vi "Drive Train Code Stuff.vi"(8 "error in (no error)":errorcluster, 11 "RobotDriveDevRef":T1) -> ()   [LabVIEW 2012]
uses:
  <vilib>/Rock Robotics/WPI/RobotDrive/WPI_RobotDriveDevRef.ctl
  <vilib>/Rock Robotics/WPI/MotorControl/WPI_MotorControlDeviceRef.ctl
  <vilib>/Rock Robotics/SystemInterfaces/Typedef/FPGA_TypedefDigitalModule.ctl
  <vilib>/Rock Robotics/SystemInterfaces/DIO/FPGA_DIOPWMChannel.ctl
  <vilib>/Rock Robotics/WPI/PWM/WPI_PWMDeadband.ctl
  <vilib>/Rock Robotics/WPI/CAN/Jaguar/SubVIs/WPI_CANJaguar_ControlMode.ctl
  <vilib>/Rock Robotics/WPI/PWM/WPI_PWMTransform_ConPane.ctl
  Robot Global Data.vi
  Documents/LabVIEW Data/No Wayne Drive/wayne drive.vi
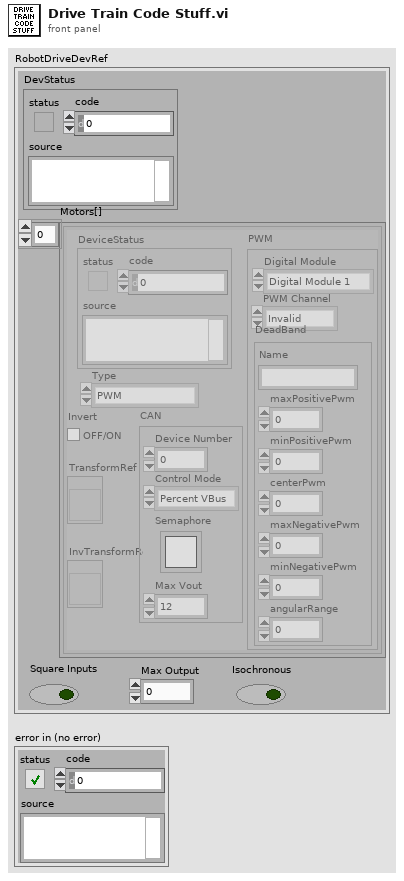
[diagram p1: front panel]
types:
  T1 = typedef "WPI_RobotDriveDevRef.ctl" = cluster{"DevStatus":errorcluster, "Motors[]":T2[], "Square Inputs":bool, "Max Output":dbl, "Isochronous":bool}
  T2 = typedef "WPI_MotorControlDeviceRef.ctl" = cluster{"DeviceStatus":errorcluster, "Type":enum16{"PWM", "CAN"}, "PWM":cluster{"Digital Module":T3, "PWM Channel":T4, "DeadBand":T5}, "CAN":cluster{"Device Number":u8, "Control Mode":T6, "Semaphore":T7, "Max Vout":dbl}, "Invert":bool, "TransformRef":T8, "InvTransformRef":T8}
  T3 = typedef "FPGA_TypedefDigitalModule.ctl" = enum16{"Digital Module 1", "Digital Module 2"}
  T4 = typedef "FPGA_DIOPWMChannel.ctl" = enum8{"PWM 1", "PWM 2", "PWM 3", "PWM 4", "PWM 5", "PWM 6", "PWM 7", "PWM 8", "PWM 9", "PWM 10", "Invalid"}
  T5 = typedef "WPI_PWMDeadband.ctl" = cluster{"Name":string, "maxPositivePwm":i32, "minPositivePwm":i32, "centerPwm":i32, "maxNegativePwm":i32, "minNegativePwm":i32, "angularRange":u16}
  T6 = typedef "WPI_CANJaguar_ControlMode.ctl" = enum8{"Percent VBus", "Current", "Speed", "Position", "Voltage"}
  T7 = typedef "Semaphore RefNum" = refnum<k1>
  T8 = typedef "WPI_PWMTransform_ConPane.ctl" = refnum<vi>
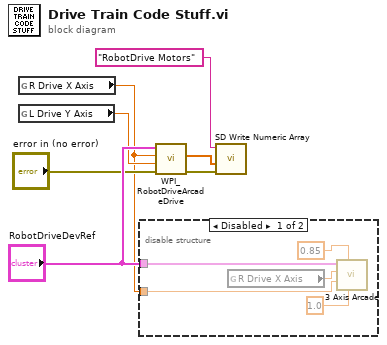
[diagram p0: block diagram]
diagram:
  n1 = global read "Robot Global Data.vi" "R Drive X Axis"() -> (w1:dbl)
  n2 = global read "Robot Global Data.vi" "L Drive Y Axis"() -> (w2:dbl)
  n3 = disable-structure shown="Disabled" {
    disable-tunnel: w1 -> [w9 _]
    disable-tunnel: "RobotDriveDevRef" -> [w8 _]
    frame Disabled {
      n4 = global read "Robot Global Data.vi" "R Drive X Axis"() -> (w10:dbl)
      n5 = call "3 Axis Arcade.vi"("Right"=1.0, "Left"=0.85, "Y axis value"=w9, "X axis value"=w10, "RobotDriveDevRef"=w8) -> ()  [unwired: 4 in, 3 out]
    }
    frame Enabled {
    }
  }
  n6 = call-poly <vilib>:"WPI_RobotDriveArcadeDrive.vi"("error in (no error)"="error in (no error)", "Y axis value"=w2, "X axis value"=w1, "RobotDriveDevRef"="RobotDriveDevRef") -> ("error out"=w3:errorcluster, "Motor Values"=w5:dbl[])  [unwired: 5 in, 1 out]
  n7 = call <vilib>:"SD Write Numeric Array.vi"("error in"=w3, "Numeric Array"=w5, "Name"="RobotDrive Motors") -> ()  [unwired: 7 in, 2 out]
